vi "hideViewerPanel.vi"(8 "error in (no error)":errorcluster, 11 "ImageStreamViewer in":refnum<class "ImageStreamViewer.lvclass">) -> (0 "error out":errorcluster, 3 "ImageStreamViewer out":refnum<class "ImageStreamViewer.lvclass">)   [LabVIEW 2011, in "Views.lvlib" / "Camera.lvlib" / "ImageStreamViewer.lvclass"]
uses:
  ImageStreamViewer.lvclass
  ImageStreamViewer.lvclass/ImageStreamViewer.ctl
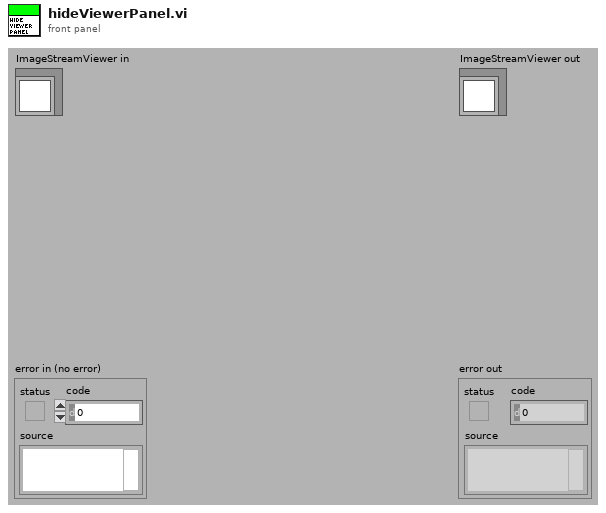
[diagram p1: front panel]
types:
  T1 = enum32{"Invalid", "Standard", "Closed", "Hidden", "Minimized", "Maximized"}
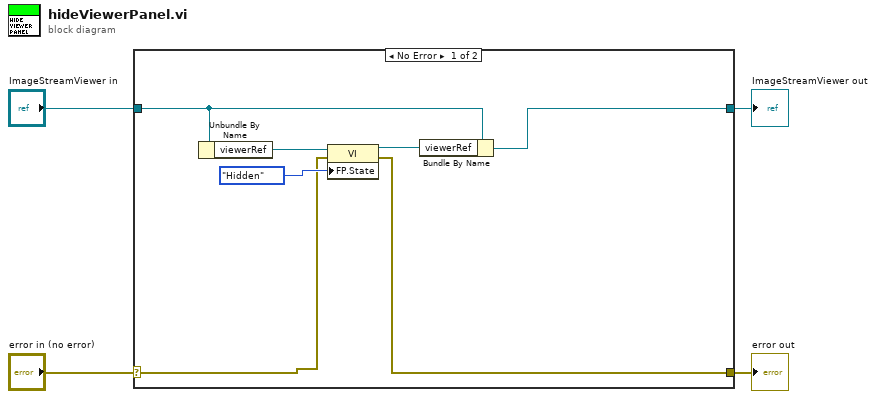
[diagram p0: block diagram]
diagram:
  n1 = case shown="No Error" "error in (no error)" {
    selector: "error in (no error)" -> [w8 w13]
    tunnel: [w7 w13] -> w3
    tunnel: [w5 w12] -> w1
    tunnel: "ImageStreamViewer in" -> [w6 w12]
    frame No Error {
      n2 = Unbundle By Name(w6) -> ("viewerRef"=w11:refnum<vi>)
      n3 = property class="VI"(reference=w11, error in=w8, "FP.State"=T1."Hidden" ("Front Panel Window:State")) -> (reference out=w9:refnum<vi>, error out=w7:errorcluster)
      n4 = Bundle By Name(cluster=w6, "viewerRef"=w9) -> (w5:refnum<class "ImageStreamViewer.lvclass">)
    }
    frame Error {
    }
  }
  "error out" <- w3
  "ImageStreamViewer out" <- w1
